vi "GET PATH.vi"() -> (3 "DB Path":path)   [LabVIEW 2020, in "DB Previtech.lvlib"]
uses:
  DB Previtech.lvlib
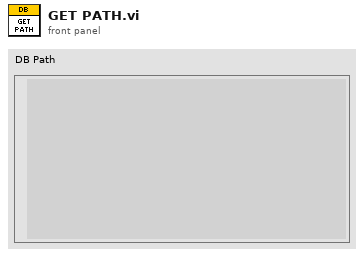
[diagram p1: front panel]
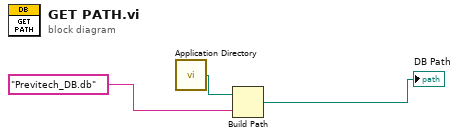
[diagram p0: block diagram]
diagram:
  n1 = call <vilib>:"Application Directory.vi"() -> ("Application Directory"=w3:path)
  n2 = Build Path(base path=w3, name or relative path="Previtech_DB.db") -> (appended path=→"DB Path":path)
